vi "action.vi"(0 "HGF_FGV_Append":refnum<class "HGF_FGV_Insert.lvclass">, 2 "Objects":refnum<class>[](array[class]), 5 "error in (no error)":errorcluster) -> (14 "dup HGF_FGV_Append":refnum<class "HGF_FGV_Insert.lvclass">, 16 "dup Objects":refnum<class>[](array[class]), 19 "error out":errorcluster)   [LabVIEW 2012, in "HGF_FGV.lvlib" / "HGF_FGV_Insert.lvclass"]
doc: "Insert object array at index."
uses:
  HGF_FGV_Insert.lvclass
  HGF_FGV_Insert.lvclass/HGF_FGV_Insert.ctl
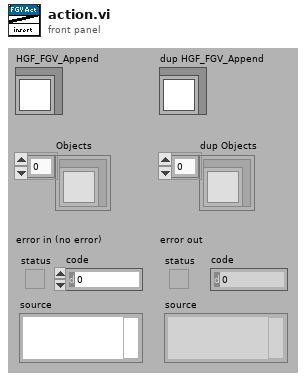
[diagram p1: front panel]
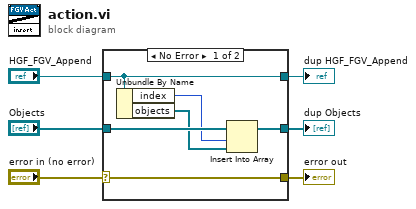
[diagram p0: block diagram]
diagram:
  n1 = case shown="No Error" "error in (no error)" {
    selector: "error in (no error)" -> [w12 w15]
    tunnel: [w12 w15] -> w5
    tunnel: [w11 w14] -> w3
    tunnel: "HGF_FGV_Append" -> [w11 w14]
    tunnel: [w9 w13] -> w2
    tunnel: "Objects" -> [w10 w13]
    frame No Error {
      n2 = Unbundle By Name(w11) -> ("index"=w7:i32, "objects"=w8:refnum<class>[])
      n3 = Insert Into Array(array=w10, index=w7, new element=w8) -> (w9:refnum<class>[])
    }
    frame Error {
    }
  }
  "error out" <- w5
  "dup HGF_FGV_Append" <- w3
  "dup Objects" <- w2
